vi "Keithley24XX_SR830_LakeShore336_4Probe_Resistance_Measurement - Two Devices.vi"() -> ()   [LabVIEW 2019]
uses:
  <instrlib>/Stanford Research 830/Public/Data/Read (All Parameters).vi
  <instrlib>/Keithley 24XX/Public/Data/Read (Single Point).vi
  <instrlib>/Keithley 24XX/Keithley 24XX.lvlib
  <instrlib>/Stanford Research 830/Stanford Research 830.lvlib
panel:
  in  "Parent Theta vs Vg 2":enum32{"XY Graph", "Waveform (Time)"}(tab)
  out "Parent Theta vs Vg : XYGraph 2":cluster{"Y":dbl[], "Y":dbl[]}[](graph)
  out "Parent: Theta vs Vg : TimeGraph 2":cluster{dbl, "Theta-Value":dbl}[](graph)
  in  "Daughter R vs Vg 2":enum32{"XY Graph", "Waveform (Time)"}(tab)
  out "Daughter Resistance vs Vg : XYGraph 2":cluster{"Y":dbl[], "Y":dbl[]}[](graph)
  out "Daughter: R vs Vg : TimeGraph 2":cluster{dbl, dbl}[](graph)
  in  "Dynamic Reserve (-1 = Auto) 3":i16(ring)=-1 items=["Auto Reserve"=-1, "High Reserve"=0, "Normal"=1, "Low Noise"=2]
  out "dup path 2":path
  in  "<File Name>.txt (Don't add extension) 2":string
  in  "Data Save Path: Daughter":path=path "C:/Users/labpc/Documents/ProbeStation Users Data"
  in  "Sensitivity (Initial Value) 2":i16(ring)=17 items=["Auto Gain"=-1, "2 nV/fA"=0, "5 nV/fA"=1, "10 nV/fA"=2, "20 nV/fA"=3, "50 nV/fA"=4, "100 nV/fA"=5, "200 nV/fA"=6, "500 nV/fA"=7, "1 uV/pA"=8, "2 uV/pA"=9, "5 uV/pA"=10, "10 uV/pA"=11, "20 uV/pA"=12, "50 uV/pA"=13, "100 uV/pA"=14, "200 uV/pA"=15, "500 uV/pA"=16, "1 mV/nA"=17, "2 mV/nA"=18, "5 mV/nA"=19, "10 mV/nA"=20, "20 mV/nA"=21, "50 mV/nA"=22, "100 mV/nA"=23, "200 mV/nA"=24, "500 mV/mA"=25, "1 V/uA"=26]
  in  "Dynamic Reserve (-1 = Auto) 2":i16(ring)=-1 items=["Auto Reserve"=-1, "High Reserve"=0, "Normal"=1, "Low Noise"=2]
  in  "Input Connection (0: Single-Ended Voltage)  2":u16(ring)=1 items=["Single-Ended Voltage", "Differential Voltage", "1 MOhm Current Gain", "100 MOhm Current Gain"]
  out "Input Coupling (0: AC) 2":u16(ring) items=["AC", "DC"]
  in  "Time Constant (8: 100ms) 2":u16(ring)=9 items=["10 us", "30 us", "100 us", "300 us", "1 ms", "3 ms", "10 ms", "30 ms", "100 ms", "300 ms", "1 s", "3 s", "10 s", "30 s", "100 s", "300 s", "1 ks", "3 ks", "10 ks", "30 ks"]
  in  "SR830 VISA resource name 2":refnum<visa-resource-name>="GPIB0::10::INSTR"
  in  "Trigger Source (0: Internal) 2":u16(ring)=1 items=["Internal", "External"]
  out "Manual Phase (0 Degree) 2":dbl
  out "Detection Harmonic Number 2":dbl=1.0
  out "External Reference Trigger (0: Sine Zero Crossing)  2":u16(ring) items=["Sine Zero Crossing", "TTL Rising Edge", "TTL Falling Edge"]
  in  "Internal Reference Frequency (1000 Hz) 2":dbl=17.0
  in  "Reference Source (1: Internal) 2":u16(ring)=1 items=["External", "Internal"]
  in  "Sine Output Amplitude (V) 2":dbl=1.0
  out "Gate\nVoltage":sgl
  out "Status":sgl
  out "Leakage \nCurrent":sgl
  out "dup path":path
  in  "<File Name>.txt (Don't add extension)":string
  in  "Data Save Path: Source":path=path "C:/Users/labpc/Documents/ProbeStation Users Data"
  in  "I_leak vs Vg":enum32{"XY Graph", "Waveform (Time)"}(tab)
  out "I_leak vs Vg : XYGraph":cluster{"Y":dbl[], "Y":dbl[]}[](graph)
  out "I_leak vs Vg : TimeGraph":cluster{dbl, "Current":sgl}[](graph)
  in  "Gate Voltage\nInitial (V)":dbl
  out "Gate Voltage\nTraversal Direction":enum16{"Upward", "Downward"}(ring)
  in  "Series Resistance \n(Apparatus Constant)":dbl=10000000.0
  in  "stop":bool
  out "Max/Min(-) \nGate Voltage (V)":dbl=80.0
  in  "Gate Voltage \nStep Size (V)":dbl=0.1
  in  "High Gate \nVoltage (V)":dbl
  in  "Low Gate \nVoltage (V)":dbl
  out "Compliance\n Level (A)":dbl=0.1
  in  "Parent Theta vs Vg":enum32{"XY Graph", "Waveform (Time)"}(tab)
  out "Parent Theta vs Vg : XYGraph":cluster{"Y":dbl[], "Y":dbl[]}[](graph)
  out "Parent: Theta vs Vg : TimeGraph":cluster{dbl, "Theta-Value":dbl}[](graph)
  in  "Parent R vs Vg":enum32{"XY Graph", "Waveform (Time)"}(tab)
  out "Parent Resistance vs Vg : XYGraph":cluster{"Y":dbl[], "Y":dbl[]}[](graph)
  out "Parent: R vs Vg : TimeGraph":cluster{dbl, dbl}[](graph)
  in  "Sensitivity (Initial Value)":i16(ring)=17 items=["Auto Gain"=-1, "2 nV/fA"=0, "5 nV/fA"=1, "10 nV/fA"=2, "20 nV/fA"=3, "50 nV/fA"=4, "100 nV/fA"=5, "200 nV/fA"=6, "500 nV/fA"=7, "1 uV/pA"=8, "2 uV/pA"=9, "5 uV/pA"=10, "10 uV/pA"=11, "20 uV/pA"=12, "50 uV/pA"=13, "100 uV/pA"=14, "200 uV/pA"=15, "500 uV/pA"=16, "1 mV/nA"=17, "2 mV/nA"=18, "5 mV/nA"=19, "10 mV/nA"=20, "20 mV/nA"=21, "50 mV/nA"=22, "100 mV/nA"=23, "200 mV/nA"=24, "500 mV/mA"=25, "1 V/uA"=26]
  in  "Dynamic Reserve (-1 = Auto)":i16(ring)=-1 items=["Auto Reserve"=-1, "High Reserve"=0, "Normal"=1, "Low Noise"=2]
  in  "Input Connection (0: Single-Ended Voltage)":u16(ring)=1 items=["Single-Ended Voltage", "Differential Voltage", "1 MOhm Current Gain", "100 MOhm Current Gain"]
  out "Input Coupling (0: AC)":u16(ring) items=["AC", "DC"]
  in  "Time Constant (8: 100ms)":u16(ring)=9 items=["10 us", "30 us", "100 us", "300 us", "1 ms", "3 ms", "10 ms", "30 ms", "100 ms", "300 ms", "1 s", "3 s", "10 s", "30 s", "100 s", "300 s", "1 ks", "3 ks", "10 ks", "30 ks"]
  in  "SR830 VISA resource name":refnum<visa-resource-name>="GPIB0::10::INSTR"
  in  "Trigger Source (0: Internal)":u16(ring) items=["Internal", "External"]
  out "Manual Phase (0 Degree)":dbl
  out "Detection Harmonic Number":dbl=1.0
  out "External Reference Trigger (0: Sine Zero Crossing)":u16(ring) items=["Sine Zero Crossing", "TTL Rising Edge", "TTL Falling Edge"]
  in  "Internal Reference Frequency (1000 Hz)":dbl=17.0
  in  "Reference Source (1: Internal)":u16(ring)=1 items=["External", "Internal"]
  in  "Sine Output Amplitude (V)":dbl=1.0
  in  "Keithley24XX VISA resource name":refnum<visa-resource-name>="GPIB0::21::INSTR" caption="Keithley 24XX VISA resource name"
  out "Internal \nMeasurement\nTime":u32
  # "MAKE SURE THE SOURCE METER IS ON TO ENSURE NO UNINTENDED JUMPS. PROGRAM WILL KEEP SOURCE METER ON ONCE RUN."
  # "SR830 Lock In Amplifier  2 - Daughter"
  # "SR830 Lock In Amplifier  1 - Sourcing"
  # "Keithley 2400 SourceMeter"
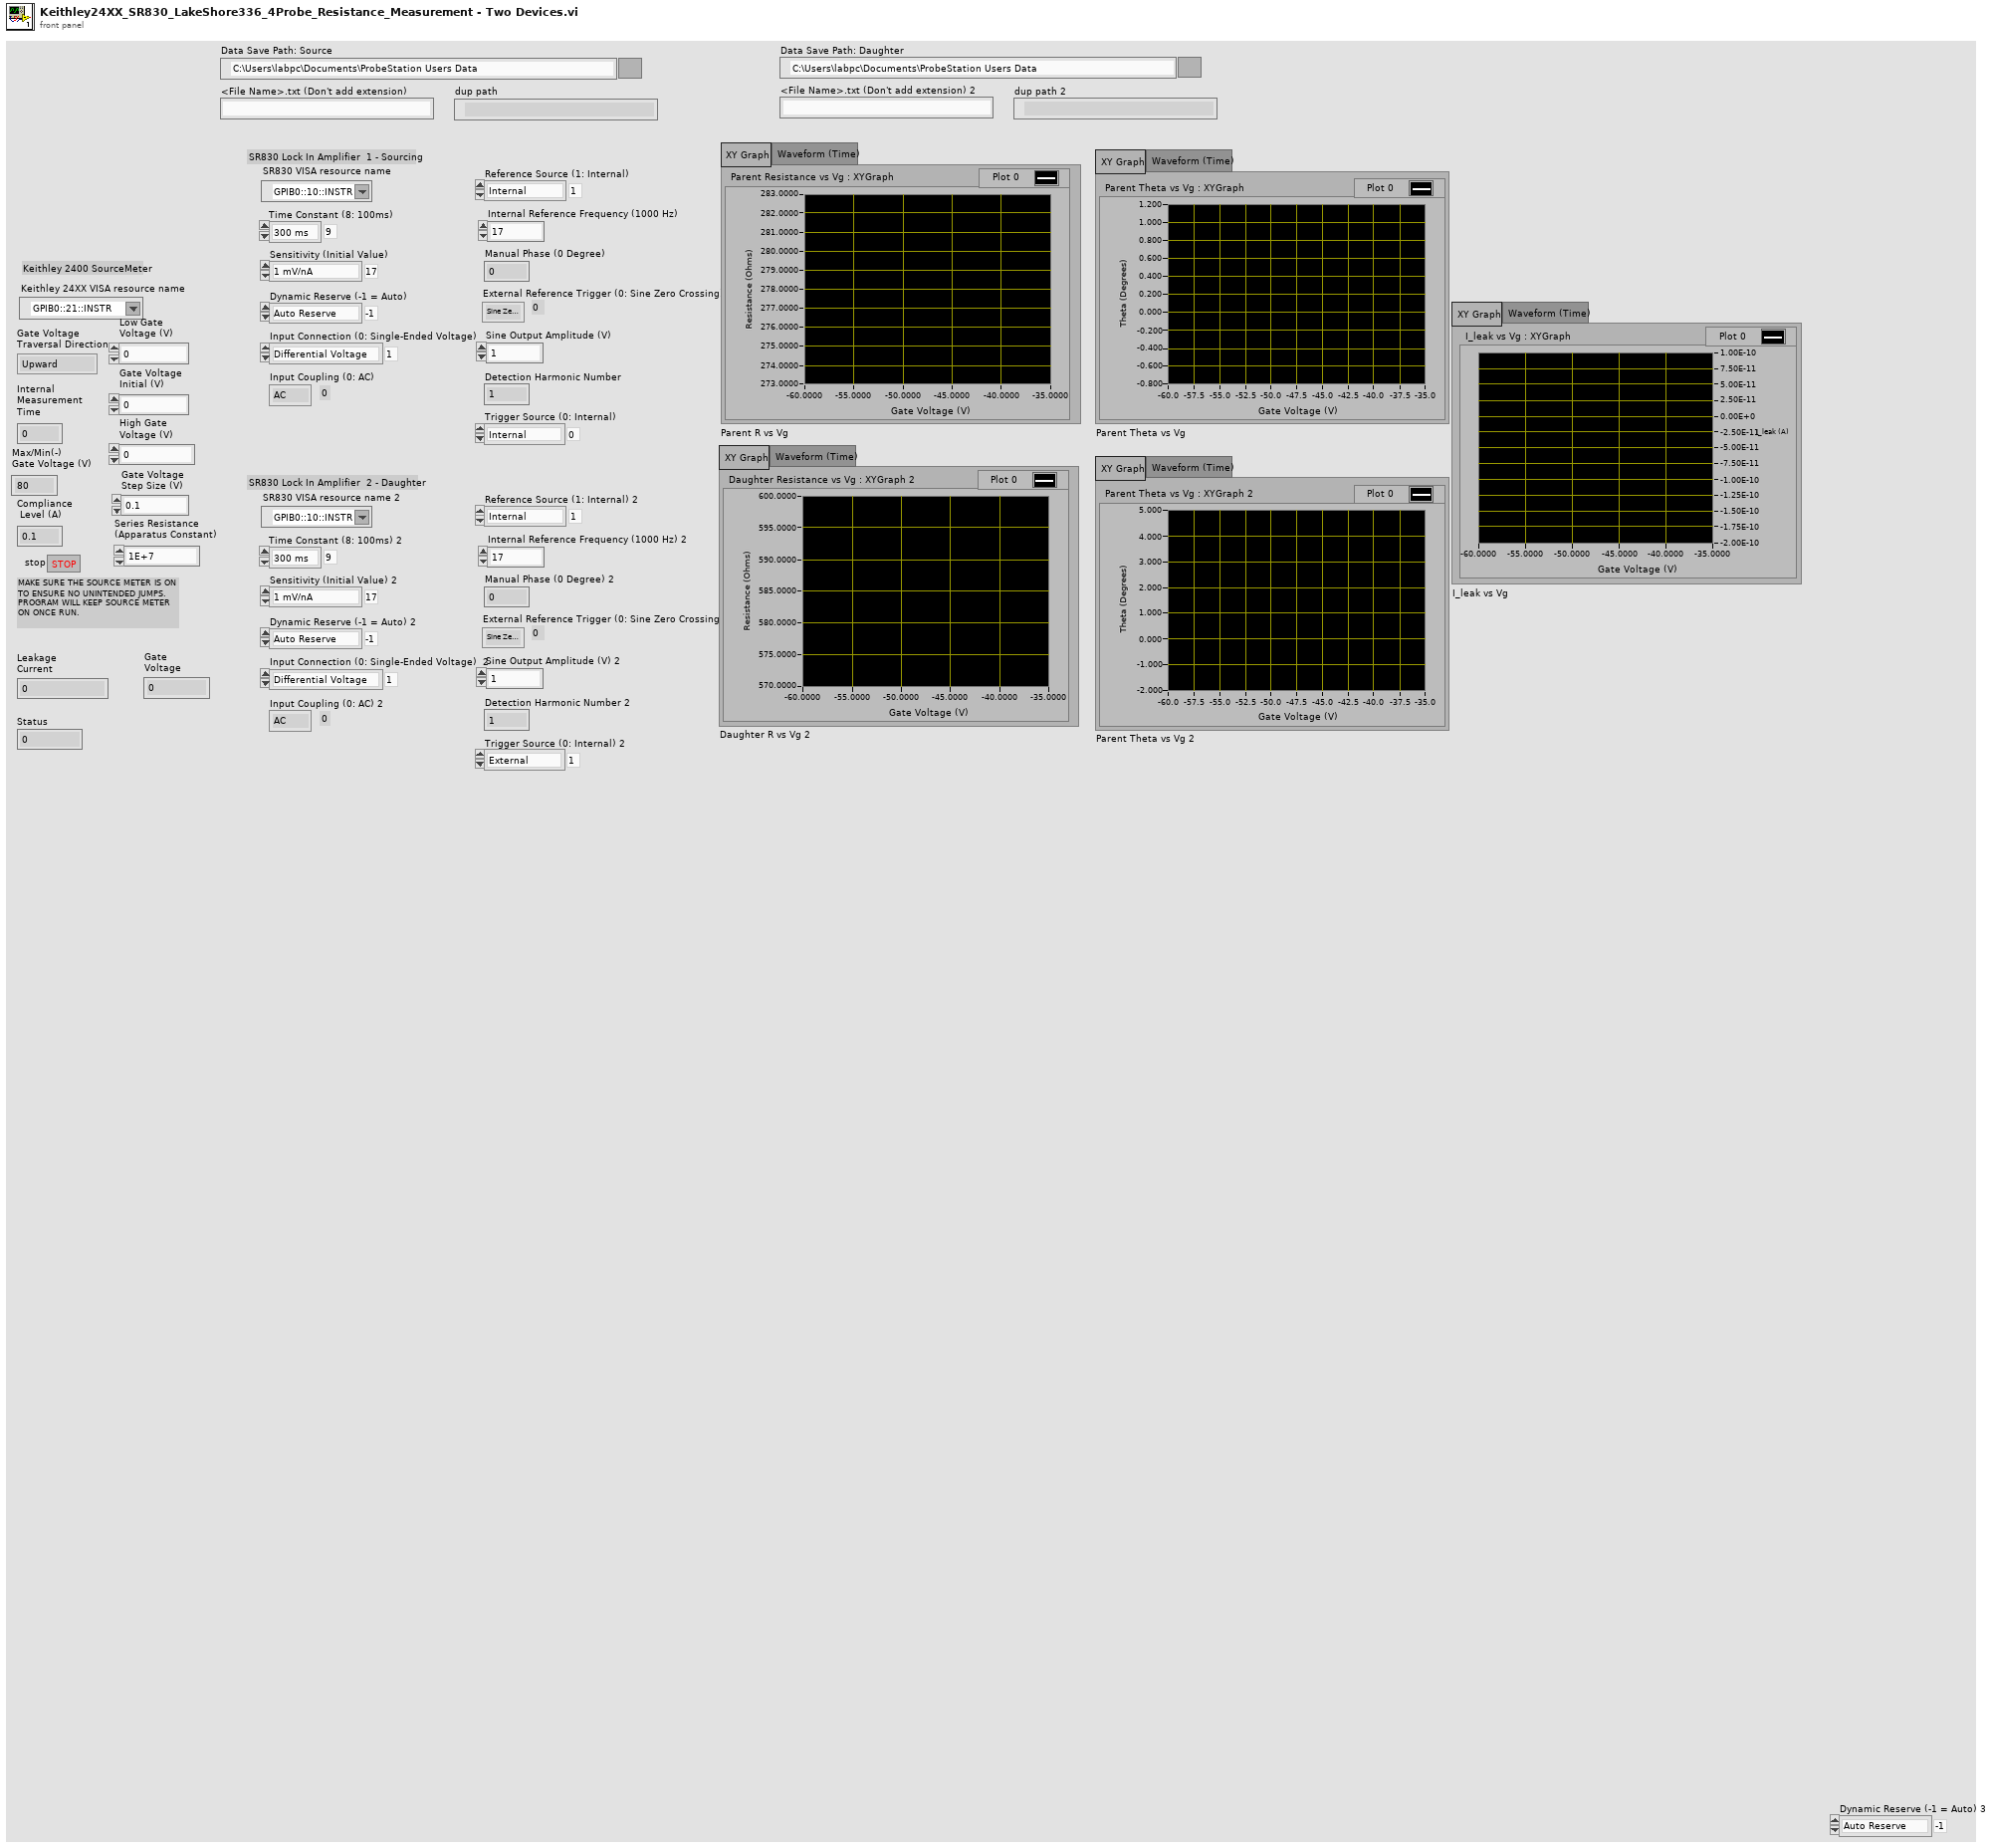
[diagram p1: front panel]
types:
  T1 = enum16{"open", "replace", "create", "open or create", "replace or create", "replace or create with confirmation"}
  T2 = cluster{"Baud Rate":u32, "Parity":u16, "Data Bits":u16, "Stop Bits":u16, "Flow Control":u16}
  T3 = cluster{"X-Value":dbl, "Y-Value":dbl, "R-Value":dbl, "Theta-Value":dbl, "Aux In 1 Value":dbl, "Aux In 2 Value":dbl, "Aux In 3 Value":dbl, "Aux In 4 Value":dbl, "Reference Frequency":dbl, "Channel 1 Display":dbl, "Channel 2 Display":dbl}
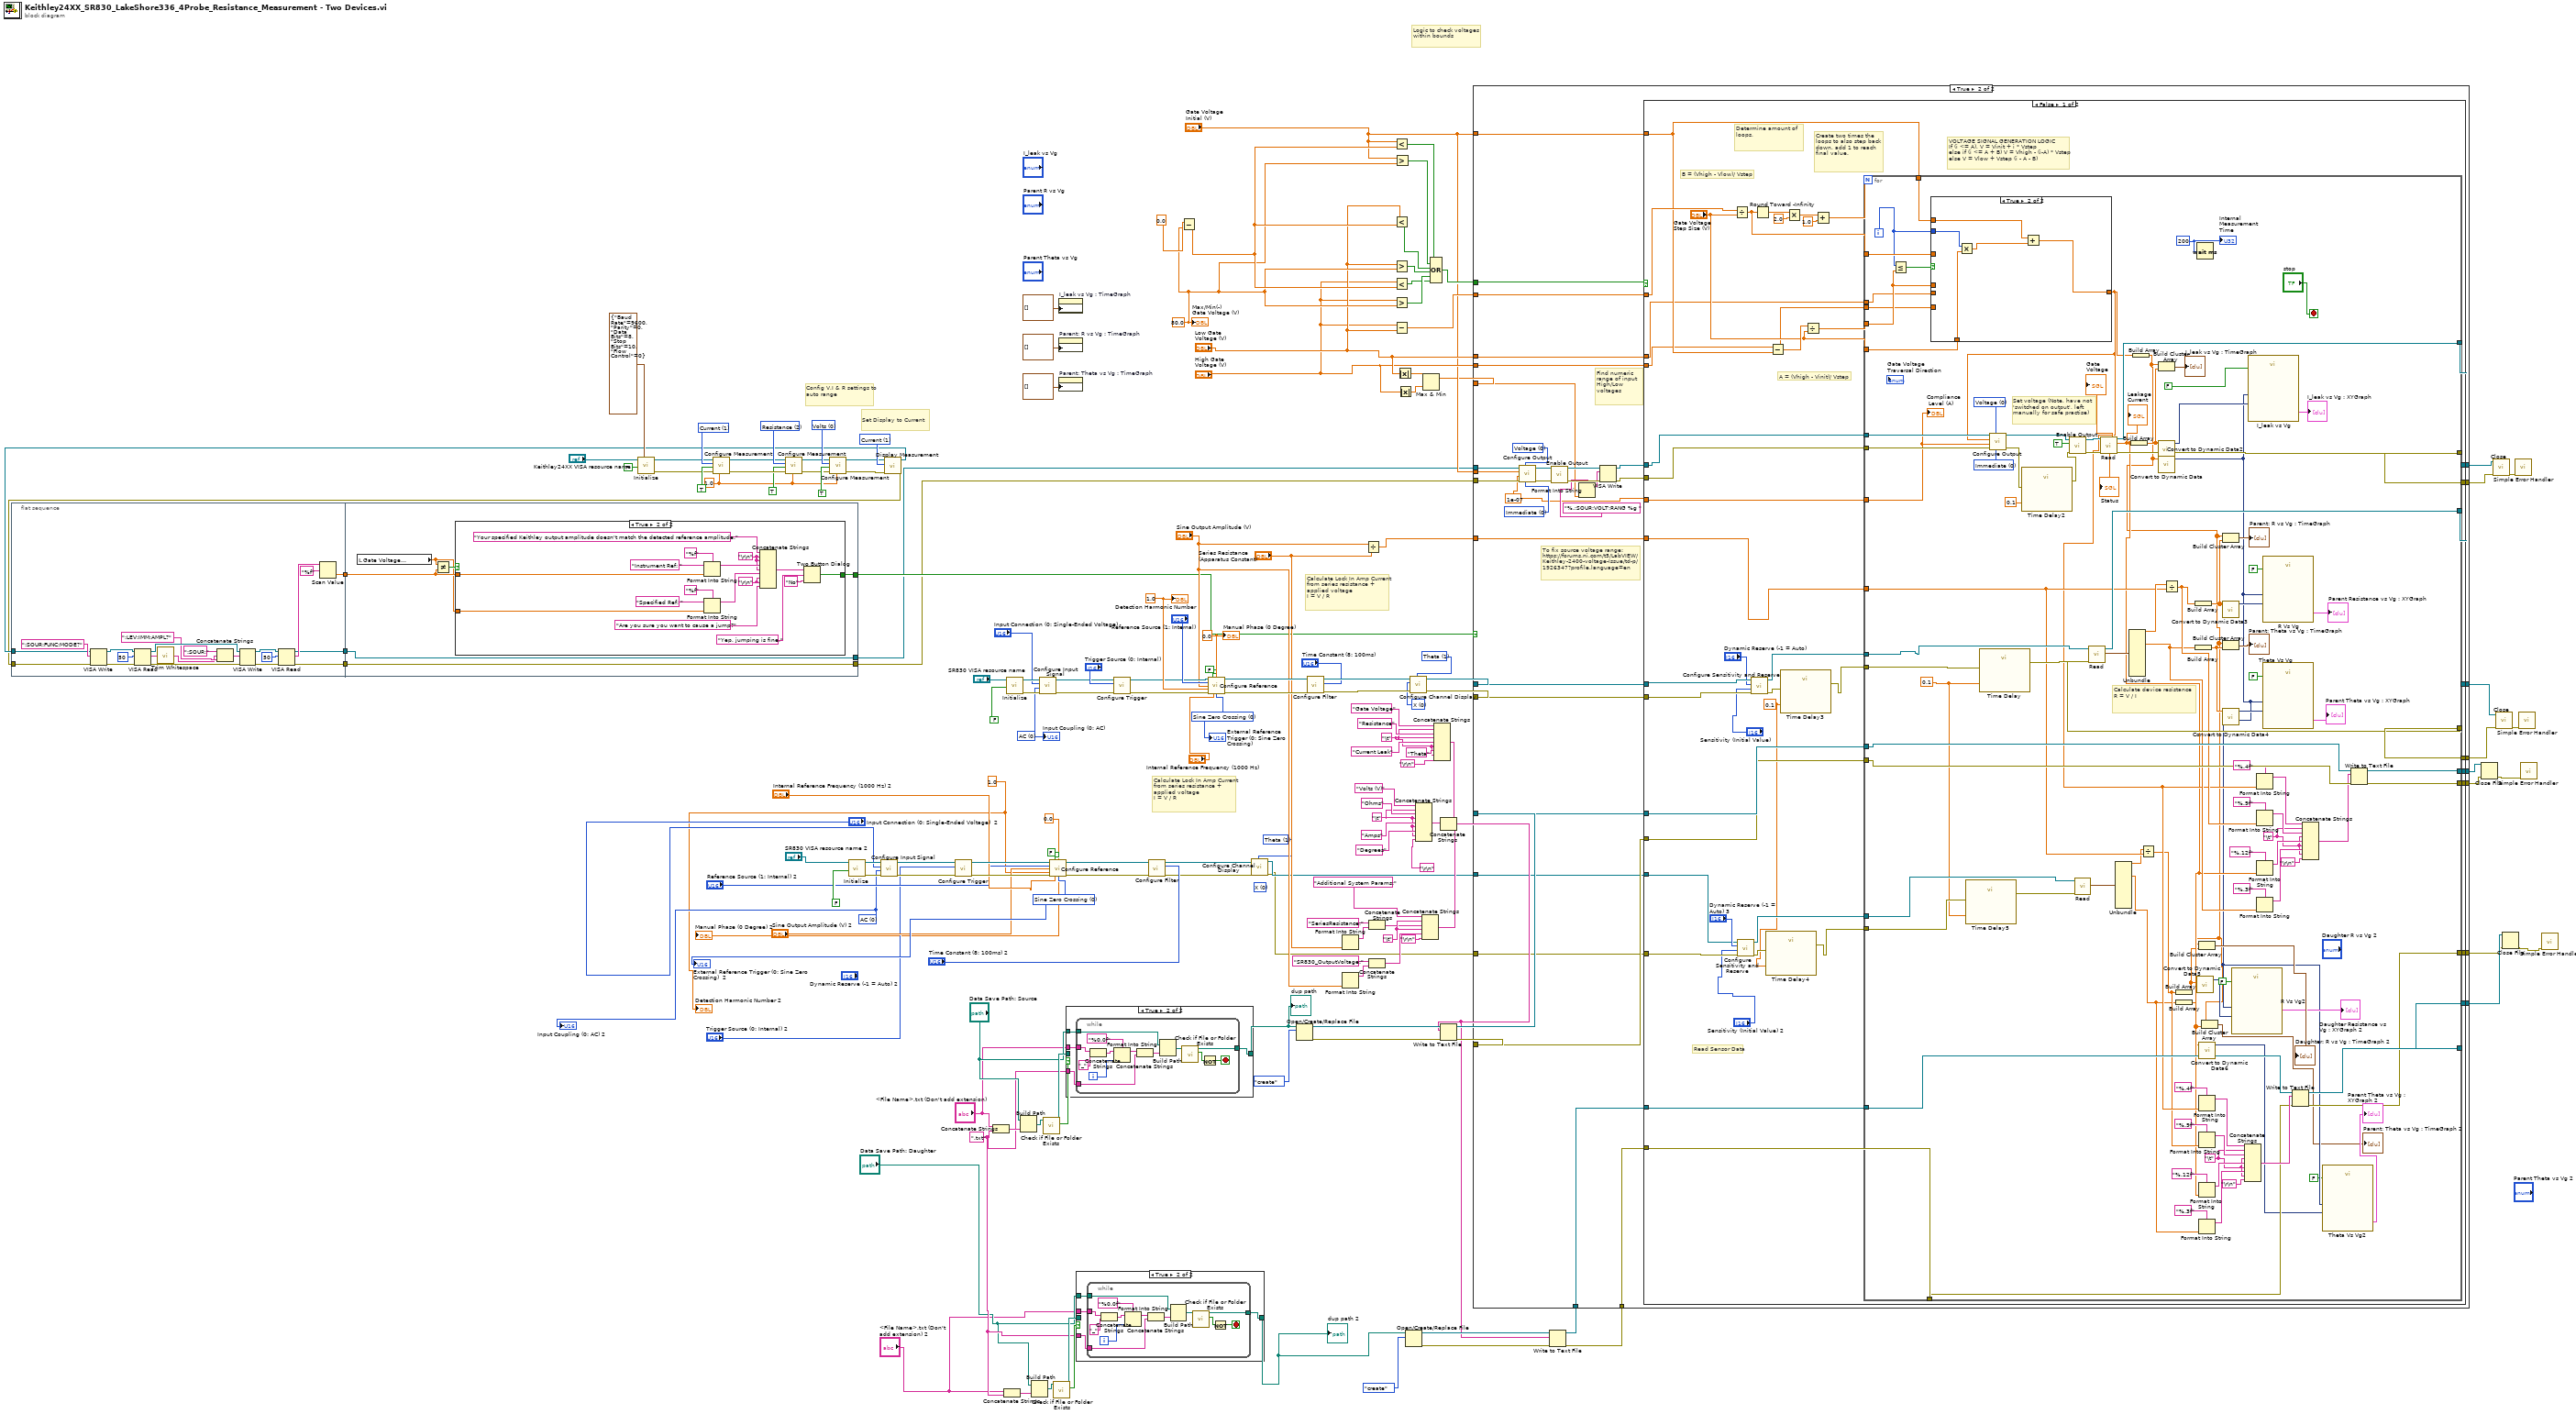
[diagram p0: block diagram]
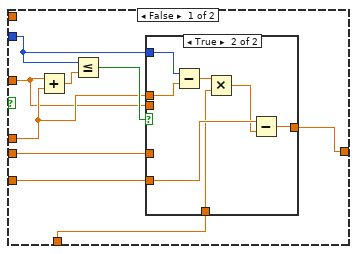
[diagram p4: hidden frame]
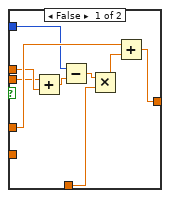
[diagram p5: hidden frame]
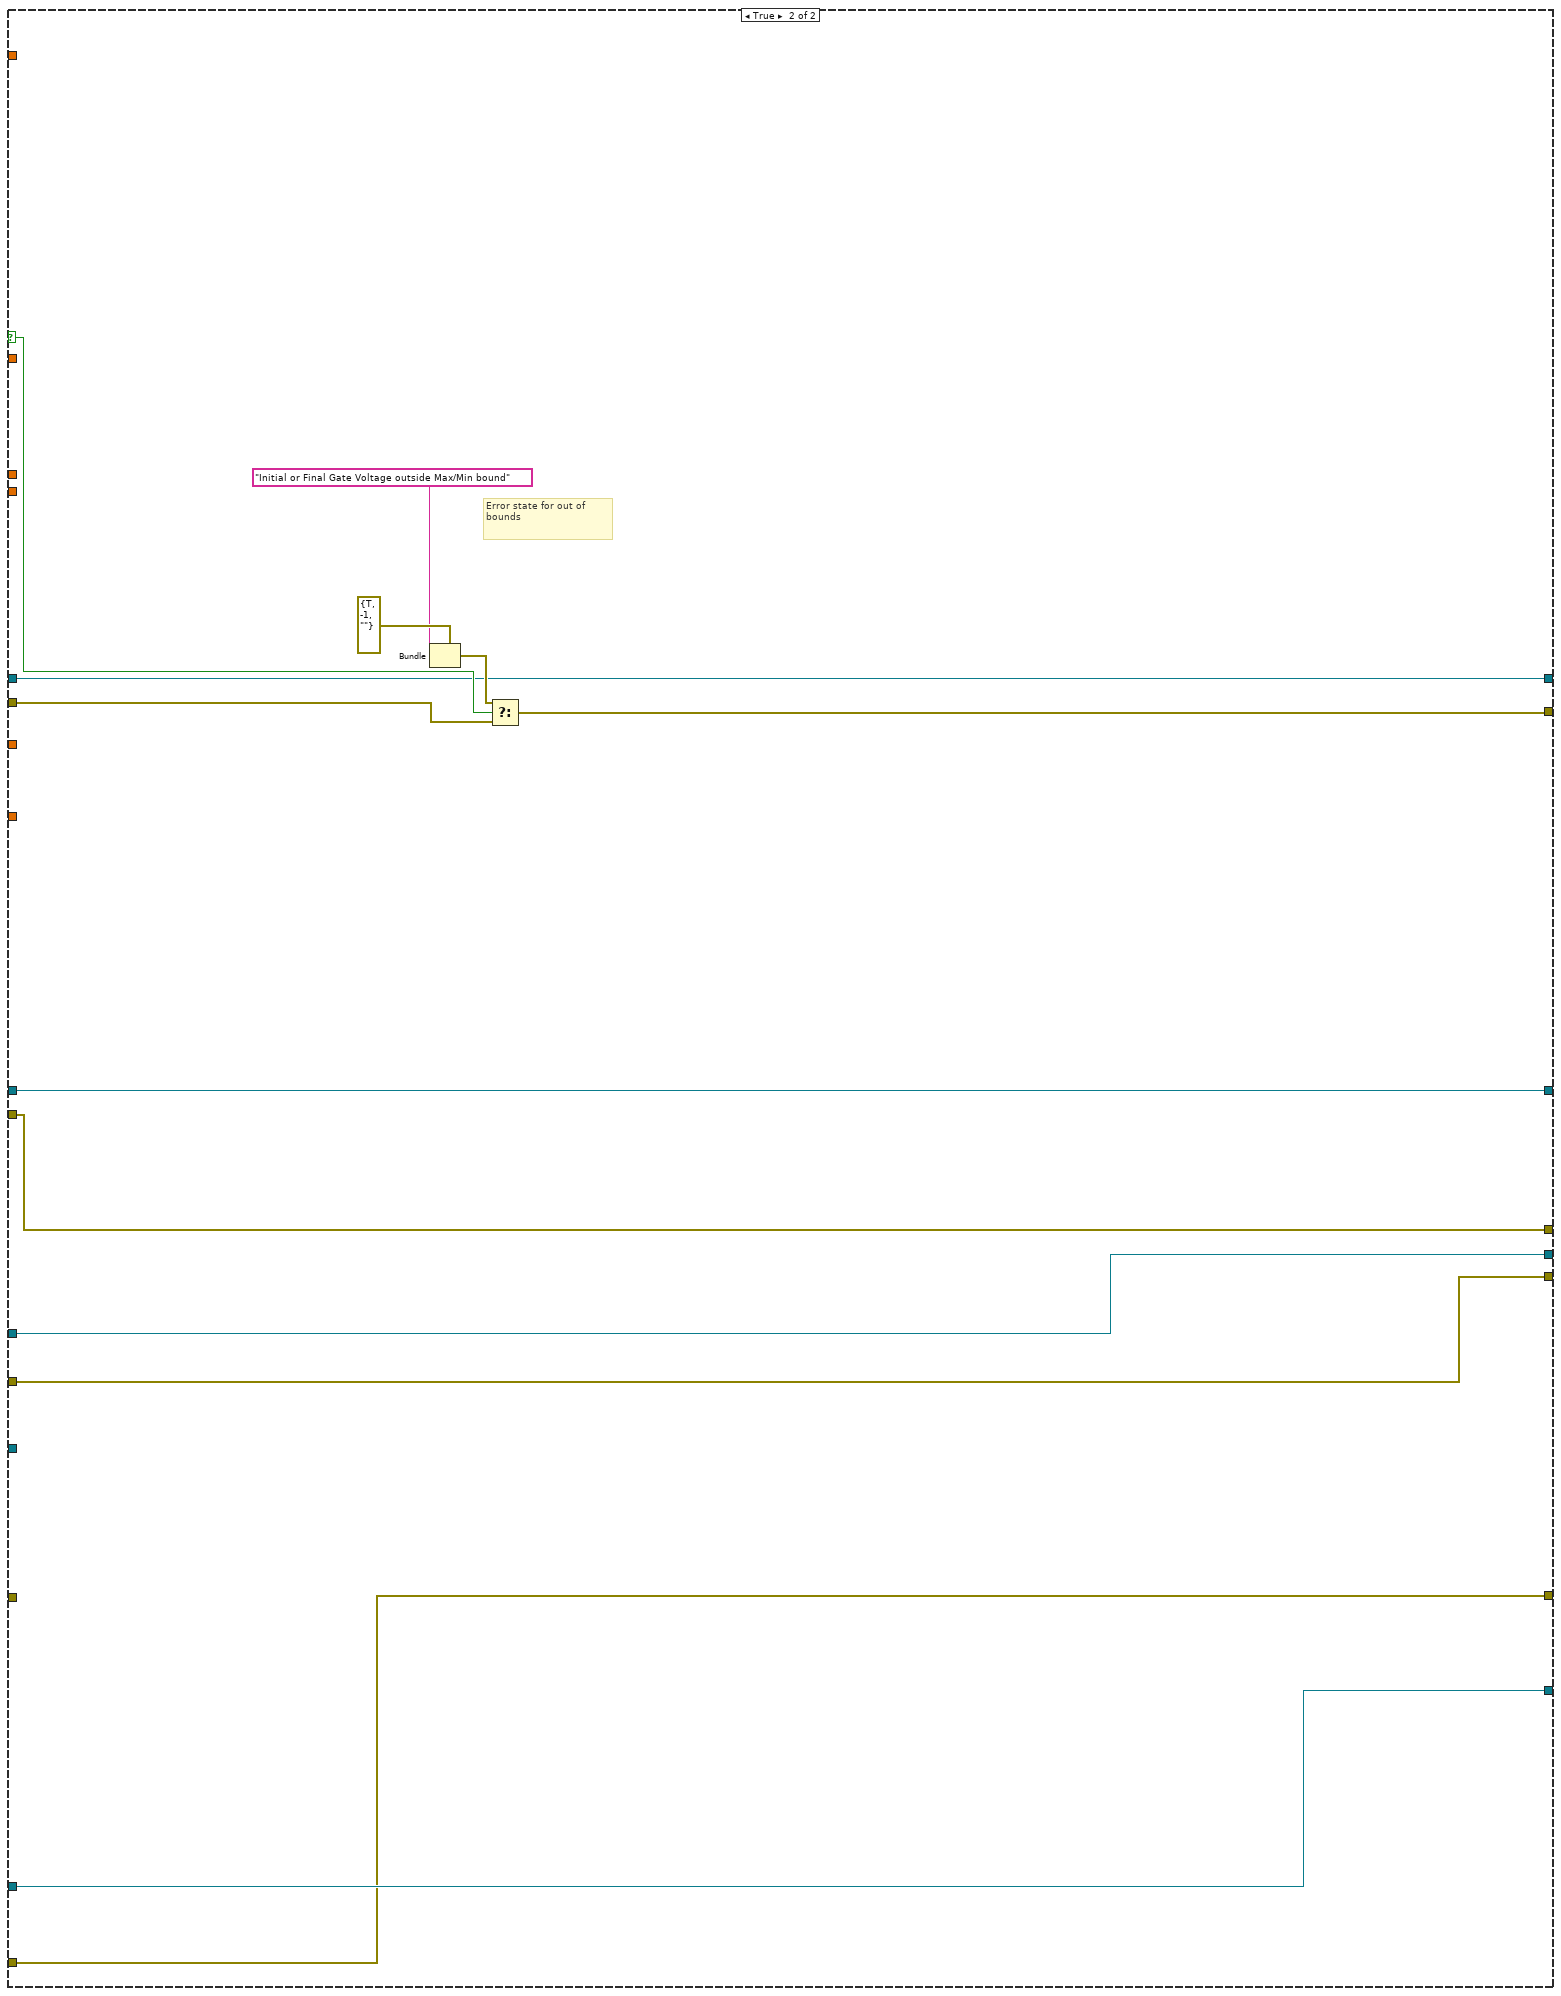
[diagram p6: hidden frame]
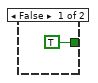
[diagram p7: hidden frame]
diagram:
  w3 = 0.0 ("Manual Phase (0 Degree)")
  w1 = 1.0 ("Detection Harmonic Number (1)")
  w17 = u16 0 items=["Sine Zero Crossing", "TTL Rising Edge", "TTL Falling Edge"] ("External Reference Trigger (0: Sine Zero Crossing)")
  w2 = u16 0 items=["AC", "DC"] ("Input Coupling (0: AC)")
  (unwired) u16 0 items=["X", "R", "X Noise", "Aux In 1", "Aux In 2"] ("Channel 1 Display (0: X)")
  w30 = u16 1 items=["Y", "Theta", "Y Noise", "Aux In 3", "Aux In 4"] ("Channel 2 Display  (0: Y)")
  w65 = "\t"
  w60 = "\t"
  w61 = "\t"
  w39 = ".txt"
  w99 = 1.0 ("Manual Range (1.0)")
  w123 = 0.0 ("Manual Phase (0 Degree)")
  w124 = 1.0 ("Detection Harmonic Number (1)")
  w125 = u16 0 items=["Sine Zero Crossing", "TTL Rising Edge", "TTL Falling Edge"] ("External Reference Trigger (0: Sine Zero Crossing)")
  w129 = u16 0 items=["AC", "DC"] ("Input Coupling (0: AC)")
  w111 = u16 0 items=["X", "R", "X Noise", "Aux In 1", "Aux In 2"] ("Channel 1 Display (0: X)")
  w139 = u16 1 items=["Y", "Theta", "Y Noise", "Aux In 3", "Aux In 4"] ("Channel 2 Display  (0: Y)")
  w144 = u16 1 items=["Voltage", "Current", "Resistance"] ("Displayed Measurement (0: Voltage)")
  w153 = u16 2 items=["Volts", "Current", "Resistance"] ("Function (0: Volts)")
  w157 = u16 1 items=["Volts", "Current", "Resistance"] ("Function (0: Volts)")
  w100 = 80.0
  w163 = u16 0 items=["Volts", "Current", "Resistance"] ("Function (0: Volts)")
  # "Calculate Lock In Amp Current from series resistance + applied voltage\nI = V / R"
  # "Logic to check voltages within bounds"
  # "Calculate Lock In Amp Current from series resistance + applied voltage\nI = V / R"
  # "Set Display to Current"
  # "Config V,I & R settings to auto range"
  n1 = flat-sequence {
    tunnel: [w167] -> w55
    tunnel: [w168] -> w54
    tunnel: [w169] -> w53
    tunnel: w52 -> [w166]
    tunnel: w51 -> [w165]
    tunnel: w55 -> [w188]
    tunnel: w54 -> [w187]
    tunnel: w53 -> [w191]
    tunnel: [w188] -> w47
    tunnel: [w187] -> w49
    tunnel: [w186] -> w50
    frame #0 {
      n2 = VISA Write(VISA resource name=w166, write buffer=":SOUR:FUNC:MODE?", error in (no error)=w165) -> (VISA resource name out=w182:refnum<visa-resource-name>, error out=w185:errorcluster)  [unwired: 1 out]
      n3 = VISA Read(VISA resource name=w182, byte count=u32 50, error in (no error)=w185) -> (VISA resource name out=w177:refnum<visa-resource-name>, read buffer=w171:string, error out=w178:errorcluster)  [unwired: 1 out]
      n4 = call <vilib>:"Trim Whitespace.vi"("string"=w171) -> ("trimmed string"=w170:string)  [unwired: 1 in]
      n5 = Concatenate Strings(":SOUR:" ("string"), w170, ":LEV:IMM:AMPL?" ("string")) -> (w174:string)
      n6 = VISA Write(VISA resource name=w177, write buffer=w174, error in (no error)=w178) -> (VISA resource name out=w179:refnum<visa-resource-name>, error out=w181:errorcluster)  [unwired: 1 out]
      n7 = VISA Read(VISA resource name=w179, byte count=u32 50, error in (no error)=w181) -> (VISA resource name out=w167:refnum<visa-resource-name>, read buffer=w172:string, error out=w168:errorcluster)  [unwired: 1 out]
      n8 = Scan Value(string=w172, format string="%f") -> (value=w169:dbl)  [unwired: 1 in, 1 out]
    }
    frame #1 {
      n9 = local read "Gate Voltage\nInitial (V)"() -> (w189:dbl)
      n10 = Not Equal?(x=w189, y=w191) -> (x != y?=w190:bool)
      n11 = case shown="True" w190 {
        tunnel: [TRUE ("T button?") w199] -> w186
        tunnel: w191 -> [_ w194]
        tunnel: w189 -> [_ w193]
        frame False {
        }
        frame True {
          w197 = "\r\n"
          w195 = "\r\n"
          n12 = Format Into String(format string="%f", initial string="Instrument Ref: ", w194) -> (resulting string=w201:string)  [unwired: 1 in, 1 out]
          n13 = Format Into String(format string="%f", initial string="Specified Ref: ", w193) -> (resulting string=w200:string)  [unwired: 1 in, 1 out]
          n14 = Concatenate Strings("Your specified Keithley output amplitude doesn't match the detected reference amplitude." ("message"), w195, w195, w201, w195, w200, w197, w197, "Are you sure you want to cause a jump?" ("string")) -> (w206:string)
          n15 = Two Button Dialog(message=w206, 1:"No" ("F button name (\"Cancel\")"), 2:"Yep, jumping is fine." ("T button name (\"OK\")")) -> (T button?=w199:bool)
        }
      }
    }
  }
  n16 = call <instrlib>:"Initialize.vi"("Serial Configuration"=T2 {"Baud Rate"=9600, "Parity"=0, "Data Bits"=8, "Stop Bits"=10, "Flow Control"=0}, "Reset (True)"=FALSE, "VISA resource name"="Keithley24XX VISA resource name") -> ("error out"=w148:errorcluster, "VISA resource name out"=w149:refnum<visa-resource-name>)  [unwired: 7 in]
  n17 = call <instrlib>:"Configure Measurement.vi"("Manual Range (1.0)"=w99, "error in (no error)"=w148, "Enable Auto Range (T:Enable)"=TRUE, "Function (0: Volts)"=w157, "VISA resource name"=w149) -> ("error out"=w155:errorcluster, "VISA resource name out"=w150:refnum<visa-resource-name>)  [unwired: 5 in]
  n18 = call <instrlib>:"Configure Measurement.vi"("Manual Range (1.0)"=w99, "error in (no error)"=w155, "Enable Auto Range (T:Enable)"=TRUE, "Function (0: Volts)"=w153, "VISA resource name"=w150) -> ("error out"=w152:errorcluster, "VISA resource name out"=w151:refnum<visa-resource-name>)  [unwired: 5 in]
  n19 = call <instrlib>:"Configure Measurement.vi"("Manual Range (1.0)"=w99, "error in (no error)"=w152, "Enable Auto Range (T:Enable)"=TRUE, "Function (0: Volts)"=w163, "VISA resource name"=w151) -> ("error out"=w142:errorcluster, "VISA resource name out"=w143:refnum<visa-resource-name>)  [unwired: 5 in]
  n20 = call <instrlib>:"Initialize.vi"("Reset (True)"=FALSE, "VISA resource name"="SR830 VISA resource name 2") -> ("error out"=w28:errorcluster, "VISA resource name out"=w29:refnum<visa-resource-name>)  [unwired: 8 in]
  n21 = call <instrlib>:"Configure Input Signal.vi"("error in (no error)"=w28, "Input Coupling (0: AC)"=w2, "Input Connection (0: Single-Ended Voltage)"="Input Connection (0: Single-Ended Voltage)  2", "VISA resource name"=w29) -> ("error out"=w24:errorcluster, "VISA resource name out"=w25:refnum<visa-resource-name>)  [unwired: 6 in]
  n22 = call <instrlib>:"Display Measurement.vi"("error in (no error)"=w142, "Displayed Measurement (0: Voltage)"=w144, "VISA resource name"=w143) -> ("error out"=w51:errorcluster, "VISA resource name out"=w52:refnum<visa-resource-name>)  [unwired: 7 in]
  n23 = call <instrlib>:"Configure Trigger.vi"("error in (no error)"=w24, "Trigger Source (0: Internal)"="Trigger Source (0: Internal) 2", "VISA resource name"=w25) -> ("error out"=w22:errorcluster, "VISA resource name out"=w23:refnum<visa-resource-name>)  [unwired: 7 in]
  n24 = Concatenate Strings("<File Name>.txt (Don't add extension)", w39) -> (w98:string)
  n25 = Concatenate Strings("<File Name>.txt (Don't add extension) 2", w39) -> (w43:string)
  n26 = call <instrlib>:"Initialize.vi"("Reset (True)"=FALSE, "VISA resource name"="SR830 VISA resource name") -> ("error out"=w136:errorcluster, "VISA resource name out"=w137:refnum<visa-resource-name>)  [unwired: 8 in]
  n27 = Build Path(base path="Data Save Path: Source", name or relative path=w98) -> (appended path=w97:path)
  n28 = Build Path(base path="Data Save Path: Daughter", name or relative path=w43) -> (appended path=w42:path)
  n29 = call <instrlib>:"Configure Input Signal.vi"("error in (no error)"=w136, "Input Coupling (0: AC)"=w129, "Input Connection (0: Single-Ended Voltage)"="Input Connection (0: Single-Ended Voltage)", "VISA resource name"=w137) -> ("error out"=w120:errorcluster, "VISA resource name out"=w121:refnum<visa-resource-name>)  [unwired: 6 in]
  n30 = call <vilib>:"Check if File or Folder Exists.vi"("path"=w97) -> ("file or folder exists?"=w96:bool, "dup path"=w95:path)  [unwired: 8 in, 1 out]
  n31 = call <instrlib>:"Configure Reference.vi"("VISA resource name"=w23, "Auto Phase (T: Enabled)"=FALSE, "Manual Phase (0 Degree)"=w3, "Reference Source (1: Internal)"="Reference Source (1: Internal) 2", "Sine Output Amplitude (1 V)"="Sine Output Amplitude (V) 2", "Detection Harmonic Number (1)"=w1, "error in (no error)"=w22, "Internal Reference Frequency (1000 Hz)"="Internal Reference Frequency (1000 Hz) 2", "External Reference Trigger (0: Sine Zero Crossing)"=w17) -> ("VISA resource name out"=w26:refnum<visa-resource-name>, "error out"=w27:errorcluster)  [unwired: 5 in]
  n32 = call <vilib>:"Check if File or Folder Exists.vi"("path"=w42) -> ("file or folder exists?"=w41:bool, "dup path"=w40:path)  [unwired: 8 in, 1 out]
  n33 = property on="I_leak vs Vg : TimeGraph" class="WFChart (strict)"("History Data"=cluster{dbl, "Current":sgl}[] []) -> ()  [unwired: 2 in, 2 out]
  n34 = property on="Parent: R vs Vg : TimeGraph" class="WFChart (strict)"("History Data"=cluster{dbl, dbl}[] []) -> ()  [unwired: 2 in, 2 out]
  n35 = property on="Parent: Theta vs Vg : TimeGraph" class="WFChart (strict)"("History Data"=cluster{dbl, "Theta-Value":dbl}[] []) -> ()  [unwired: 2 in, 2 out]
  n36 = case shown="True" w96 {
    tunnel: [w209 w210] -> w90
    tunnel: w95 -> [w209 _]
    tunnel: "Data Save Path: Source" -> [_ w211]
    tunnel: "<File Name>.txt (Don't add extension)" -> [_ w213]
    tunnel: w39 -> [_ w212]
    frame False {
    }
    frame True {
      n37 = while {
        tunnel: w213 -> [w216]
        tunnel: w212 -> [w221]
        tunnel: w211 -> [w219]
        tunnel: [w217] -> w210
        i -> [w223]
        stop <- w225 stop-if-true
        n38 = Concatenate Strings(w216, "_" ("string")) -> (w215:string)
        n39 = Format Into String(format string="%0.0f", initial string=w215, w223) -> (resulting string=w222:string)  [unwired: 1 in, 1 out]
        n40 = Concatenate Strings(w222, w221) -> (w220:string)
        n41 = Build Path(base path=w219, name or relative path=w220) -> (appended path=w218:path)
        n42 = call <vilib>:"Check if File or Folder Exists.vi"("path"=w218) -> ("file or folder exists?"=w226:bool, "dup path"=w217:path)  [unwired: 8 in, 1 out]
        n43 = Not(x=w226) -> (.not. x?=w225:bool)
      }
    }
  }
  "dup path" <- w90
  n44 = case shown="True" w41 {
    tunnel: [w227 w228] -> w33
    tunnel: w40 -> [w227 _]
    tunnel: "Data Save Path: Daughter" -> [_ w229]
    tunnel: "<File Name>.txt (Don't add extension) 2" -> [_ w231]
    tunnel: w39 -> [_ w230]
    frame False {
    }
    frame True {
      n45 = while {
        tunnel: w231 -> [w234]
        tunnel: w230 -> [w239]
        tunnel: w229 -> [w237]
        tunnel: [w235] -> w228
        i -> [w241]
        stop <- w243 stop-if-true
        n46 = Concatenate Strings(w234, "_" ("string")) -> (w233:string)
        n47 = Format Into String(format string="%0.0f", initial string=w233, w241) -> (resulting string=w240:string)  [unwired: 1 in, 1 out]
        n48 = Concatenate Strings(w240, w239) -> (w238:string)
        n49 = Build Path(base path=w237, name or relative path=w238) -> (appended path=w236:path)
        n50 = call <vilib>:"Check if File or Folder Exists.vi"("path"=w236) -> ("file or folder exists?"=w244:bool, "dup path"=w235:path)  [unwired: 8 in, 1 out]
        n51 = Not(x=w244) -> (.not. x?=w243:bool)
      }
    }
  }
  "dup path 2" <- w33
  n52 = call <instrlib>:"Configure Trigger.vi"("error in (no error)"=w120, "Trigger Source (0: Internal)"="Trigger Source (0: Internal)", "VISA resource name"=w121) -> ("error out"=w118:errorcluster, "VISA resource name out"=w119:refnum<visa-resource-name>)  [unwired: 7 in]
  n53 = call <instrlib>:"Configure Filter.vi"("error in (no error)"=w27, "Time Constant (8: 100ms)"="Time Constant (8: 100ms) 2", "VISA resource name"=w26) -> ("error out"=w10:errorcluster, "VISA resource name out"=w11:refnum<visa-resource-name>)  [unwired: 7 in]
  n54 = Subtract(x=0.0, y=w100) -> (x-y=w105:dbl)
  n55 = call <instrlib>:"Configure Reference.vi"("VISA resource name"=w119, "Auto Phase (T: Enabled)"=FALSE, "Manual Phase (0 Degree)"=w123, "Reference Source (1: Internal)"="Reference Source (1: Internal)", "Sine Output Amplitude (1 V)"="Sine Output Amplitude (V)", "Detection Harmonic Number (1)"=w124, "error in (no error)"=w118, "Internal Reference Frequency (1000 Hz)"="Internal Reference Frequency (1000 Hz)", "External Reference Trigger (0: Sine Zero Crossing)"=w125) -> ("VISA resource name out"=w126:refnum<visa-resource-name>, "error out"=w127:errorcluster)  [unwired: 5 in]
  n56 = call <instrlib>:"Configure Channel Display.vi"("Channel 2 Display  (0: Y)"=w30, "error in (no error)"=w10, "VISA resource name"=w11) -> ("error out"=w8:errorcluster, "VISA resource name out"=w9:refnum<visa-resource-name>)  [unwired: 7 in]
  n57 = Open/Create/Replace File(file path (use dialog)=w90, operation (0:open)=T1."create") -> (refnum out=w91:refnum<file>, error out=w89:errorcluster)  [unwired: 4 in, 1 out]
  n58 = call <instrlib>:"Configure Filter.vi"("error in (no error)"=w127, "Time Constant (8: 100ms)"="Time Constant (8: 100ms)", "VISA resource name"=w126) -> ("error out"=w146:errorcluster, "VISA resource name out"=w145:refnum<visa-resource-name>)  [unwired: 7 in]
  n59 = Format Into String("Series Resistance \n(Apparatus Constant)") -> (resulting string=w83:string)  [unwired: 3 in, 1 out]
  n60 = Format Into String("Sine Output Amplitude (V)") -> (resulting string=w82:string)  [unwired: 3 in, 1 out]
  n61 = Divide(x="Sine Output Amplitude (V)", y="Series Resistance \n(Apparatus Constant)") -> (x/y=w117:dbl)
  n62 = Concatenate Strings("SeriesResistance:" ("string"), w83) -> (w64:string)
  n63 = Concatenate Strings("SR830_OutputVoltage:" ("string"), w82) -> (w63:string)
  n64 = Less?(x="Gate Voltage\nInitial (V)", y=w105) -> (x < y?=w103:bool)
  n65 = Less?(x="Low Gate \nVoltage (V)", y=w105) -> (x < y?=w109:bool)
  n66 = Greater?(x="Low Gate \nVoltage (V)", y=w100) -> (0:w108:bool)
  n67 = Less?(x="High Gate \nVoltage (V)", y=w105) -> (x < y?=w106:bool)
  n68 = Greater?(x="High Gate \nVoltage (V)", y=w100) -> (0:w107:bool)
  n69 = Subtract(x="High Gate \nVoltage (V)", y="Low Gate \nVoltage (V)") -> (x-y=w101:dbl)
  n70 = Greater?(x="Gate Voltage\nInitial (V)", y=w100) -> (0:w104:bool)
  n71 = Absolute Value(x="Low Gate \nVoltage (V)") -> (abs(x)=w59:dbl)
  n72 = Absolute Value(x="High Gate \nVoltage (V)") -> (abs(x)=w58:dbl)
  n73 = Open/Create/Replace File(file path (use dialog)=w33, operation (0:open)=T1."create") -> (refnum out=w35:refnum<file>, error out=w34:errorcluster)  [unwired: 4 in, 1 out]
  n74 = call <instrlib>:"Configure Channel Display.vi"("Channel 2 Display  (0: Y)"=w139, "error in (no error)"=w146, "Channel 1 Display (0: X)"=w111, "VISA resource name"=w145) -> ("error out"=w134:errorcluster, "VISA resource name out"=w135:refnum<visa-resource-name>)  [unwired: 6 in]
  n75 = Concatenate Strings("Volts (V)" ("string"), w60, "Ohms" ("string"), w60, "Amps" ("string"), w60, "Degrees" ("string"), w60, "\r\n") -> (w76:string)
  n76 = Concatenate Strings("Additional System Params:" ("string"), w65, w64, w65, w63, "\r\n") -> (w66:string)
  n77 = Max & Min(x=w59, y=w58) -> (max(x,y)=w46:dbl)  [unwired: 1 out]
  n78 = Compound Arithmetic op=OR(w103, w104, w109, w108, w107, w106) -> (w102:bool)
  n79 = Concatenate Strings("Gate Voltage" ("string"), w61, "Resistance" ("string"), w61, "Current Leak" ("string"), w61, "Theta" ("string"), w61, "\r\n") -> (w77:string)
  n80 = Concatenate Strings(w77, w76, w66) -> (w32:string)
  n81 = Write to Text File(file (use dialog)=w91, text=w32, error in=w89) -> (refnum out=w87:refnum<file>, error out=w86:errorcluster)  [unwired: 1 in, 1 out]
  n82 = Write to Text File(file (use dialog)=w35, text=w32, error in=w34) -> (refnum out=w15:refnum<file>, error out=w13:errorcluster)  [unwired: 1 in, 1 out]
  n83 = case shown="True" w50 {
    tunnel: [w252 w289] -> w161
    tunnel: [w251 w288] -> w160
    tunnel: w135 -> [w250 w287]
    tunnel: w134 -> [w249 w286]
    tunnel: [w250 w285] -> w133
    tunnel: [w249 w284] -> w132
    tunnel: w117 -> [_ w283]
    tunnel: w102 -> [_ w282]
    tunnel: w101 -> [_ w281]
    tunnel: w87 -> [w248 w280]
    tunnel: w86 -> [w247 w279]
    tunnel: [w248 w278] -> w85
    tunnel: [w247 w277] -> w84
    tunnel: "Low Gate \nVoltage (V)" -> [_ w276]
    tunnel: "High Gate \nVoltage (V)" -> [_ w275]
    tunnel: "Gate Voltage\nInitial (V)" -> [_ w274]
    tunnel: w49 -> [w251 w266]
    tunnel: "Gate Voltage\nInitial (V)" -> [_ w265]
    tunnel: w47 -> [w252 w264]
    tunnel: w46 -> [_ w262]
    tunnel: [w246 w258] -> w16
    tunnel: w15 -> [w246 w257]
    tunnel: [w245 w256] -> w14
    tunnel: w13 -> [w245 w255]
    tunnel: w9 -> [_ w254]
    tunnel: w8 -> [_ w253]
    frame False {
    }
    frame True {
      w268 = u16 0 items=["Immediate", "Triggered"] ("Output Type  (0: Immediate)")
      w261 = 1e-07 ("Compliance  Level (0.1)")
      w267 = u16 0 items=["Voltage", "Current"] ("Source Mode  (0: Voltage)")
      # "Find numeric range of input High/Low voltages"
      # "To fix source voltage range:\nhttps://forums.ni.com/t5/LabVIEW/Keithley-2400-voltage-Issue/td-p/1926347?profile.language=en"
      n84 = call <instrlib>:"Configure Output.vi"("Output Type  (0: Immediate)"=w268, "Source Mode  (0: Voltage)"=w267, "error in (no error)"=w266, "Compliance  Level (0.1)"=w261, "Output Level (0)"=w265, "VISA resource name"=w264) -> ("error out"=w273:errorcluster, "VISA resource name out"=w272:refnum<visa-resource-name>)  [unwired: 4 in]
      n85 = call <instrlib>:"Enable Output.vi"("error in (no error)"=w273, "VISA resource name"=w272) -> ("error out"=w271:errorcluster, "VISA resource name out"=w270:refnum<visa-resource-name>)  [unwired: 8 in]
      n86 = Format Into String(format string="%.;SOUR:VOLT:RANG %g ", w262) -> (resulting string=w269:string)  [unwired: 2 in, 1 out]
      n87 = VISA Write(VISA resource name=w270, write buffer=w269, error in (no error)=w271) -> (VISA resource name out=w259:refnum<visa-resource-name>, error out=w260:errorcluster)  [unwired: 1 out]
      n88 = case shown="False" w282 {
        selector: w282 -> [_ w479]
        tunnel: w260 -> [w333 w478]
        tunnel: w259 -> [w303 w473]
        tunnel: [w332 w473] -> w289
        tunnel: [w331 w474] -> w288
        tunnel: w287 -> [w326 w472]
        tunnel: w286 -> [w327 w471]
        tunnel: [w329 w472] -> w285
        tunnel: [w328 w471] -> w284
        tunnel: w283 -> [w323 _]
        tunnel: w281 -> [w318 _]
        tunnel: w276 -> [w311 _]
        tunnel: w275 -> [w312 _]
        tunnel: w274 -> [w314 _]
        tunnel: w280 -> [w308 w470]
        tunnel: w279 -> [w307 w469]
        tunnel: [w306 w470] -> w278
        tunnel: [w305 w469] -> w277
        tunnel: w261 -> [w302 _]
        tunnel: [w301 w468] -> w258
        tunnel: w257 -> [w300 w468]
        tunnel: [w299 w467] -> w256
        tunnel: w255 -> [w298 w467]
        tunnel: w254 -> [w295 _]
        tunnel: w253 -> [w294 _]
        frame False {
          w290 = 0.1 ("Delay Time (s)")
          # "Read Sensor Data"
          # "VOLTAGE SIGNAL GENERATION LOGIC\nIf (i <= A), V = Vinit + i * Vstep\nelse if (i <= A + B) V = Vhigh - (i-A) * Vstep\nelse V = Vlow + Vstep (i - A - B)"
          # "B = (Vhigh - Vlow)/ Vstep"
          # "A = (Vhigh - Vinit)/ Vstep"
          # "Create two times the loops to also step back down, add 1 to reach final value."
          # "Determine amount of loops,"
          n89 = Divide(x=w318, y="Gate Voltage \nStep Size (V)") -> (x/y=w313:dbl)
          n90 = call <instrlib>:"Configure Sensitivity and Reserve.vi"("error in (no error)"=w294, "Sensitivity (-1: Auto gain)"="Sensitivity (Initial Value) 2", "Dynamic Reserve (-1: Auto Reserve)"="Dynamic Reserve (-1 = Auto) 3", "VISA resource name"=w295) -> ("error out"=w296:errorcluster, "VISA resource name out"=w293:refnum<visa-resource-name>)  [unwired: 6 in]
          n91 = call <instrlib>:"Configure Sensitivity and Reserve.vi"("error in (no error)"=w327, "Sensitivity (-1: Auto gain)"="Sensitivity (Initial Value)", "Dynamic Reserve (-1: Auto Reserve)"="Dynamic Reserve (-1 = Auto)", "VISA resource name"=w326) -> ("error out"=w309:errorcluster, "VISA resource name out"=w325:refnum<visa-resource-name>)  [unwired: 6 in]
          n92 = Round Toward -Infinity(1:w313) -> (0:w321:dbl)
          n93 = call "Time Delay4"("error in (no error)"=w296, "Delay Time (s)"=w290) -> ("error out"=w292:errorcluster)  [unwired: 9 in]
          n94 = Subtract(x=w312, y=w314) -> (x-y=w317:dbl)
          n95 = call "Time Delay3"("error in (no error)"=w309, "Delay Time (s)"=w290) -> ("error out"=w310:errorcluster)  [unwired: 9 in]
          n96 = Multiply(x=w321, y=2.0) -> (x*y=w320:dbl)
          n97 = Divide(x=w317, y="Gate Voltage \nStep Size (V)") -> (x/y=w315:dbl)
          n98 = Add(x=w320, y=1.0) -> (x+y=w319:dbl)
          n99 = for {
            N: w319 -> [_]
            tunnel: w303 -> [w432]
            tunnel: w333 -> [w398]
            tunnel: [w436] -> w332
            tunnel: [w435] -> w331
            tunnel: [w425] -> w329
            tunnel: [w426] -> w328
            tunnel: w325 -> [w380]
            tunnel: w310 -> [w381]
            tunnel: w323 -> [w367]
            tunnel: "Gate Voltage \nStep Size (V)" -> [w404]
            tunnel: w315 -> [w402]
            tunnel: w314 -> [w405]
            tunnel: w313 -> [w403]
            tunnel: w312 -> [w401]
            tunnel: w311 -> [w400]
            tunnel: w308 -> [w395]
            tunnel: w307 -> [w394]
            tunnel: [w393] -> w306
            tunnel: [w392] -> w305
            tunnel: w302 -> [w374]
            tunnel: [w353] -> w301
            tunnel: w300 -> [w354]
            tunnel: [w351] -> w299
            tunnel: w298 -> [w352]
            tunnel: w293 -> [w370]
            tunnel: w292 -> [w369]
            i -> [w379]
            stop <- "stop" stop-if-true
            w356 = "\t"
            w377 = "\t"
            w399 = u16 0 items=["Immediate", "Triggered"] ("Output Type  (0: Immediate)")
            w368 = 0.1 ("Delay Time (s)")
            w433 = u32 200 ("milliseconds to wait")
            w428 = u16 0 items=["Voltage", "Current"] ("Source Mode  (0: Voltage)")
            # "Calculate device resistance\nR = V / I"
            # "Set voltage (Note, have not 'switched on output', left manually for safe practise)"
            n100 = Less Or Equal?(x=w379, y=w402) -> (x <= y?=w406:bool)
            n101 = case shown="True" w406 {
              tunnel: [w443 w462] -> w350
              tunnel: w405 -> [_ w465]
              tunnel: w379 -> [w440 w466]
              tunnel: w404 -> [w441 w463]
              tunnel: w403 -> [w437 _]
              tunnel: w402 -> [w439 _]
              tunnel: w401 -> [w442 _]
              tunnel: w400 -> [w438 _]
              frame False {
                n102 = Add(x=w437, y=w439) -> (x+y=w444:dbl)
                n103 = Less Or Equal?(x=w440, y=w444) -> (x <= y?=w445:bool)
                n104 = case shown="True" w445 {
                  tunnel: [w451 w460] -> w443
                  tunnel: w442 -> [_ w461]
                  tunnel: w441 -> [w453 w458]
                  tunnel: w440 -> [w448 w457]
                  tunnel: w439 -> [w447 w456]
                  tunnel: w438 -> [w454 _]
                  tunnel: w437 -> [w446 _]
                  frame False {
                    n105 = Add(x=w446, y=w447) -> (x+y=w449:dbl)
                    n106 = Subtract(x=w448, y=w449) -> (x-y=w450:dbl)
                    n107 = Multiply(x=w450, y=w453) -> (x*y=w452:dbl)
                    n108 = Add(x=w454, y=w452) -> (x+y=w451:dbl)
                  }
                  frame True {
                    n109 = Subtract(x=w457, y=w456) -> (x-y=w459:dbl)
                    n110 = Multiply(x=w459, y=w458) -> (x*y=w455:dbl)
                    n111 = Subtract(x=w461, y=w455) -> (x-y=w460:dbl)
                  }
                }
              }
              frame True {
                n112 = Multiply(x=w466, y=w463) -> (x*y=w464:dbl)
                n113 = Add(x=w465, y=w464) -> (x+y=w462:dbl)
              }
            }
            n114 = call "Time Delay5"("error in (no error)"=w369, "Delay Time (s)"=w368) -> ("error out"=w371:errorcluster)  [unwired: 9 in]
            n115 = call "Time Delay"("error in (no error)"=w381, "Delay Time (s)"=w368) -> ("error out"=w422:errorcluster)  [unwired: 9 in]
            n116 = call <instrlib>:"Configure Output.vi"("Output Type  (0: Immediate)"=w399, "Source Mode  (0: Voltage)"=w428, "error in (no error)"=w398, "Compliance  Level (0.1)"=w374, "Output Level (0)"=w350, "VISA resource name"=w432) -> ("error out"=w397:errorcluster, "VISA resource name out"=w431:refnum<visa-resource-name>)  [unwired: 4 in]
            n117 = call "Time Delay2"("error in (no error)"=w397, "Delay Time (s)"=0.1) -> ("error out"=w396:errorcluster)  [unwired: 9 in]
            n118 = call <instrlib>:"Enable Output.vi"("error in (no error)"=w396, "Enable Output (T: Enable)"=TRUE, "VISA resource name"=w431) -> ("error out"=w430:errorcluster, "VISA resource name out"=w429:refnum<visa-resource-name>)  [unwired: 7 in]
            n119 = call-poly <instrlib>:"Read.vi"("error in (no error)"=w371, "VISA resource name"=w370) -> ("Parameter Values"=w372:T3)  [unwired: 7 in, 2 out]
            n120 = call-poly <instrlib>:"Read.vi"("error in (no error)"=w422, "VISA resource name"=w380) -> ("error out"=w426:errorcluster, "Parameter Values"=w424:T3, "VISA resource name out"=w425:refnum<visa-resource-name>)  [unwired: 7 in]
            n121 = call-poly <instrlib>:"Read.vi"("VISA resource name"=w429, "error in (no error)"=w430) -> ("Voltage"=→"Gate\nVoltage":sgl, "VISA resource name out"=w436:refnum<visa-resource-name>, "Current"=w347:sgl, "Status"=→"Status":sgl, "error out"=w435:errorcluster)  [unwired: 7 in, 2 out]
            "Leakage \nCurrent" <- w347
            n122 = Unbundle(w372) -> ("X-Value"=w366:dbl, "Theta-Value"=w348:dbl)  [unwired: 9 out]
            n123 = Unbundle(w424) -> ("X-Value"=w423:dbl, "Theta-Value"=w385:dbl)  [unwired: 9 out]
            n124 = Build Array(w347) -> (w419:sgl[])
            n125 = Build Array(w350) -> (w339:dbl[])
            n126 = Divide(x=w366, y=w367) -> (x/y=w349:dbl)
            n127 = Build Cluster Array(w339, w419) -> (→"I_leak vs Vg : TimeGraph":cluster{dbl, "Current":sgl}[])
            n128 = call "Convert to Dynamic Data2"("Array"=w419) -> ("Dynamic Data Type"=w418:dynamicdata)  [unwired: 3 in]
            n129 = call "Convert to Dynamic Data"("Array"=w339) -> ("Dynamic Data Type"=w342:dynamicdata)  [unwired: 3 in]
            n130 = Divide(x=w423, y=w367) -> (x/y=w386:dbl)
            n131 = Build Array(w349) -> (w344:dbl[])
            n132 = Build Array(w348) -> (w338:dbl[])
            n133 = Build Array(w386) -> (w417:dbl[])
            n134 = Build Array(w385) -> (w415:dbl[])
            n135 = Wait (ms)(milliseconds to wait=w433) -> ()  [unwired: 1 out]
            n136 = call "Convert to Dynamic Data5"("Array"=w344) -> ("Dynamic Data Type"=w343:dynamicdata)  [unwired: 3 in]
            n137 = Format Into String(format string="%.4f", w350) -> (resulting string=w365:string)  [unwired: 2 in, 1 out]
            n138 = Format Into String(format string="%.9f", w349) -> (resulting string=w364:string)  [unwired: 2 in, 1 out]
            n139 = Format Into String(format string="%.12f", w347) -> (resulting string=w363:string)  [unwired: 2 in, 1 out]
            n140 = Format Into String(format string="%.3f", w348) -> (resulting string=w362:string)  [unwired: 2 in, 1 out]
            n141 = Build Cluster Array(w339, w344) -> (→"Daughter: R vs Vg : TimeGraph 2":cluster{dbl, dbl}[])
            n142 = call "Convert to Dynamic Data6"("Array"=w338) -> ("Dynamic Data Type"=w341:dynamicdata)  [unwired: 3 in]
            n143 = Build Cluster Array(w339, w338) -> (→"Parent: Theta vs Vg : TimeGraph 2":cluster{dbl, "Theta-Value":dbl}[])
            n144 = Build Cluster Array(w339, w417) -> (→"Parent: R vs Vg : TimeGraph":cluster{dbl, dbl}[])
            n145 = call "Convert to Dynamic Data3"("Array"=w417) -> ("Dynamic Data Type"=w416:dynamicdata)  [unwired: 3 in]
            n146 = Build Cluster Array(w339, w415) -> (→"Parent: Theta vs Vg : TimeGraph":cluster{dbl, "Theta-Value":dbl}[])
            n147 = call "Convert to Dynamic Data4"("Array"=w415) -> ("Dynamic Data Type"=w414:dynamicdata)  [unwired: 3 in]
            n148 = call "R Vs Vg2"("Reset"=FALSE, "Y Input"=w343, "X Input"=w342) -> ("XY Graph"=→"Daughter Resistance vs Vg : XYGraph 2":cluster{"X":dbl[], "Y":dbl[]}[])  [unwired: 7 in, 1 out]
            n149 = Concatenate Strings(w365, w356, w364, w356, w363, w356, w362, w356, "\r\n") -> (w361:string)
            n150 = call "I_leak vs Vg"("Reset"=FALSE, "Y Input"=w418, "X Input"=w342) -> ("XY Graph"=→"I_leak vs Vg : XYGraph":cluster{"X":dbl[], "Y":dbl[]}[])  [unwired: 7 in, 1 out]
            n151 = Format Into String(format string="%.4f", w350) -> (resulting string=w391:string)  [unwired: 2 in, 1 out]
            n152 = Format Into String(format string="%.9f", w386) -> (resulting string=w390:string)  [unwired: 2 in, 1 out]
            n153 = Format Into String(format string="%.12f", w347) -> (resulting string=w389:string)  [unwired: 2 in, 1 out]
            n154 = Format Into String(format string="%.3f", w385) -> (resulting string=w388:string)  [unwired: 2 in, 1 out]
            n155 = call "R Vs Vg"("Reset"=FALSE, "Y Input"=w416, "X Input"=w342) -> ("XY Graph"=→"Parent Resistance vs Vg : XYGraph":cluster{"X":dbl[], "Y":dbl[]}[])  [unwired: 7 in, 1 out]
            n156 = call "Theta Vs Vg"("Reset"=FALSE, "Y Input"=w414, "X Input"=w342) -> ("XY Graph"=→"Parent Theta vs Vg : XYGraph":cluster{"X":dbl[], "Y":dbl[]}[])  [unwired: 7 in, 1 out]
            n157 = Write to Text File(file (use dialog)=w354, text=w361, error in=w352) -> (refnum out=w353:refnum<file>, error out=w351:errorcluster)  [unwired: 1 in, 1 out]
            n158 = Concatenate Strings(w391, w377, w390, w377, w389, w377, w388, w377, "\r\n") -> (w387:string)
            n159 = call "Theta Vs Vg2"("Reset"=FALSE, "Y Input"=w341, "X Input"=w342) -> ("XY Graph"=→"Parent Theta vs Vg : XYGraph 2":cluster{"X":dbl[], "Y":dbl[]}[])  [unwired: 7 in, 1 out]
            n160 = Write to Text File(file (use dialog)=w395, text=w387, error in=w394) -> (refnum out=w393:refnum<file>, error out=w392:errorcluster)  [unwired: 1 in, 1 out]
            "Compliance\n Level (A)" <- w374
            "Internal \nMeasurement\nTime" <- w433
          }
        }
        frame True {
          # "Error state for out of bounds"
          n161 = Bundle(cluster=errorcluster {"status"=TRUE, "code"=-1, "source"=""} ("error constant"), "source"="Initial or Final Gate Voltage outside Max/Min bound") -> (w475:errorcluster)  [unwired: 2 in]
          n162 = Select(t=w475, s=w479, f=w478) -> (s? t:f=w474:errorcluster)
        }
      }
    }
  }
  n163 = Close File(refnum=w85, error in=w84) -> (error out=w88:errorcluster)  [unwired: 1 out]
  n164 = call <instrlib>:"Close.vi"("error in (no error)"=w160, "VISA resource name"=w161) -> ("error out"=w159:errorcluster)  [unwired: 9 in]
  n165 = call <instrlib>:"Close.vi"("error in (no error)"=w132, "VISA resource name"=w133) -> ("error out"=w147:errorcluster)  [unwired: 9 in]
  n166 = Close File(refnum=w16, error in=w14) -> (error out=w12:errorcluster)  [unwired: 1 out]
  n167 = call <vilib>:"Simple Error Handler.vi"("error in (no error)"=w159) -> ()  [unwired: 4 in, 5 out]
  n168 = call <vilib>:"Simple Error Handler.vi"("error in (no error)"=w147) -> ()  [unwired: 4 in, 5 out]
  n169 = call <vilib>:"Simple Error Handler.vi"("error in (no error)"=w88) -> ()  [unwired: 4 in, 5 out]
  n170 = call <vilib>:"Simple Error Handler.vi"("error in (no error)"=w12) -> ()  [unwired: 4 in, 5 out]
  "Max/Min(-) \nGate Voltage (V)" <- w100
  "Input Coupling (0: AC)" <- w129
  "External Reference Trigger (0: Sine Zero Crossing)" <- w125
  "Detection Harmonic Number" <- w124
  "Manual Phase (0 Degree)" <- w123
  "Manual Phase (0 Degree) 2" <- w3
  "Detection Harmonic Number 2" <- w1
  "External Reference Trigger (0: Sine Zero Crossing)  2" <- w17
  "Input Coupling (0: AC) 2" <- w2
